vi "EmptyMenu.vi"(8 "error in (no error)":errorcluster, 11 "Menu in":refnum<class "MGI_ToolStrip.lvclass">) -> (0 "error out":errorcluster, 3 "Menu out":refnum<class "MGI_ToolStrip.lvclass">)   [LabVIEW 2019, in "MGI_ToolStrip.lvclass"]
doc: "Removes all menu items from the menu.\n\nAuthored by Derek E. Trepanier\nsupport@mooregoodideas.com\nwww.mooregoodideas.com\n\nCopyright (c) 2012, Moore Good Ideas, Inc.\n\nAll rights reserved.\n\nRedistribution and use in source and binary forms, with or without modification, are permitted provided that the following conditions are met:\n\n * Redistributions of source code must retain the above copyright notice, this list of conditions and the following disclaimer.\n * Redistributions in binary form must reproduce the above copyright notice, this list of conditions and the following disclaimer in the documentation and/or other materials provided with the distribution.\n * Neither the name of Moore Good Ideas, Inc. nor the names of its contributors may be used to endorse or promote products derived from this software without specific prior written permission.\n\nTHIS SOFTWARE IS PROVIDED BY THE COPYRIGHT HOLDERS AND CONTRIBUTORS \"AS IS\" AND ANY EXPRESS OR IMPLIED WARRANTIES, INCLUDING, BUT NOT LIMITED TO, THE IMPLIED WARRANTIES OF MERCHANTABILITY AND FITNESS FOR A PARTICULAR PURPOSE ARE DISCLAIMED. IN NO EVENT SHALL THE COPYRIGHT OWNER OR CONTRIBUTORS BE LIABLE FOR ANY DIRECT, INDIRECT, INCIDENTAL, SPECIAL, EXEMPLARY, OR CONSEQUENTIAL DAMAGES (INCLUDING, BUT NOT LIMITED TO, PROCUREMENT OF SUBSTITUTE GOODS OR SERVICES; LOSS OF USE, DATA, OR PROFITS; OR BUSINESS INTERRUPTION) HOWEVER CAUSED AND ON ANY THEORY OF LIABILITY, WHETHER IN CONTRACT, STRICT LIABILITY, OR TORT (INCLUDING NEGLIGENCE OR OTHERWISE) ARISING IN ANY WAY OUT OF THE USE OF THIS SOFTWARE, EVEN IF ADVISED OF THE POSSIBILITY OF SUCH DAMAGE."
uses:
  MGI_ToolStrip.lvclass
  MGI_ToolStrip.lvclass/MGI_ToolStrip.ctl
  System.Windows.Forms
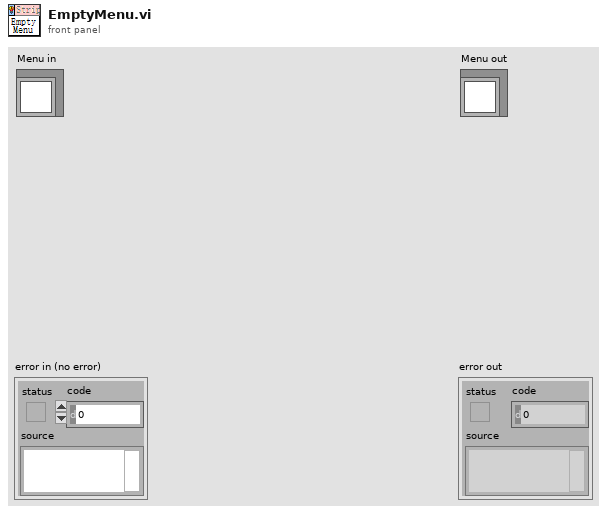
[diagram p1: front panel]
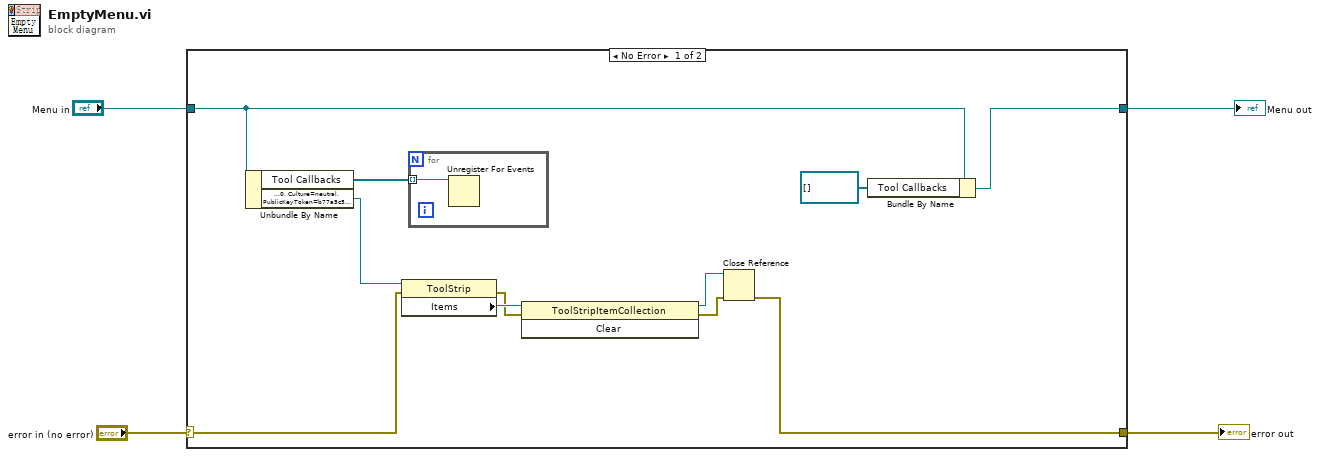
[diagram p0: block diagram]
diagram:
  n1 = case shown="No Error" "error in (no error)" {
    selector: "error in (no error)" -> [w11 w18]
    tunnel: [w8 w18] -> w1
    tunnel: [w6 w17] -> w3
    tunnel: "Menu in" -> [w7 w17]
    frame No Error {
      n2 = Unbundle By Name(w7) -> ("Tool Callbacks"=w15:refnum<k27>[], "ToolStrip"=w12:refnum<k24>)
      n3 = property class="ToolStrip"(reference=w12, error in=w11) -> (error out=w13:errorcluster, "Items"=w14:refnum<k24>)  [unwired: 1 out]
      n4 = for {
        tunnel: w15 -> [w16] mode=indexing
        n5 = Unregister For Events(event registration refnum=w16) -> ()  [unwired: 1 in, 1 out]
      }
      n6 = invoke class="ToolStripItemCollection" method="Clear"(reference=w14, error in=w13) -> (reference out=w10:refnum<k24>, error out=w9:errorcluster)  [unwired: 1 in, 1 out]
      n7 = Close Reference(reference=w10, error in (no error)=w9) -> (error out=w8:errorcluster)
      n8 = Bundle By Name(cluster=w7, "Tool Callbacks"=refnum<k27>[] []) -> (w6:refnum<class "MGI_ToolStrip.lvclass">)
    }
    frame Error {
    }
  }
  "error out" <- w1
  "Menu out" <- w3
